vi "Resize Image (Scale).vi"(7 "Filter (Default)":T1, 8 "error in (no error)":errorcluster, 10 "Scale":dbl=1.0, 11 "Image":T2) -> (0 "error out":errorcluster, 3 "Resized Image":T2)   [LabVIEW 2020, in "G-Image.lvlib"]
doc: "Resize the input image by the specified scale multiplier.\n\n<b>Filter</b> sets the filter type used when resizing. When set to Default, the Catmull-Rom filter is used when upsampling images, and the Mitchell filter used when downsampling images.\n\n<b>Note:</b> 8-bit images will be converted to true color images when resized."
uses:
  G-Image.lvlib
  <vilib>/picture/picture.llb/imagedata.ctl
  Controls/Resize Filter.ctl
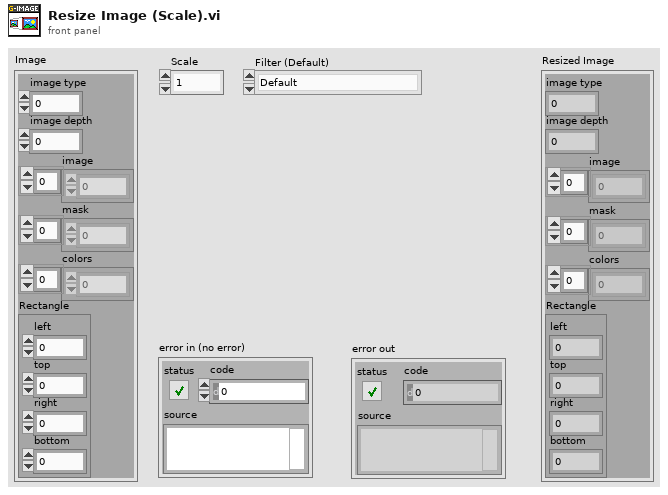
[diagram p1: front panel]
types:
  T1 = typedef "G-Image.lvlib/Resize Filter.ctl" = enum16{"Default", "Box", "Triangle", "Cubic B-Spline", "Catmull-Rom", "Mitchell"}
  T2 = typedef "imagedata.ctl" = cluster{"image type":i32, "image depth":i32, "image":u8[], "mask":u8[], "colors":u32[], "Rectangle":cluster{"left":i16, "top":i16, "right":i16, "bottom":i16}}
  T3 = cluster{"left":i16, "top":i16, "right":i16, "bottom":i16}
  T4 = cluster{"left":dbl, "top":dbl, "right":dbl, "bottom":dbl}
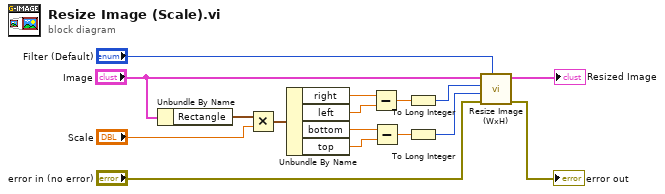
[diagram p0: block diagram]
diagram:
  n1 = Unbundle By Name("Image") -> ("Rectangle"=w16:T3)
  n2 = Multiply(x=w16, y="Scale") -> (x*y=w14:T4)
  n3 = Unbundle By Name(w14) -> ("right"=w13:dbl, "left"=w12:dbl, "bottom"=w9:dbl, "top"=w8:dbl)
  n4 = Subtract(x=w13, y=w12) -> (x-y=w11:dbl)
  n5 = Subtract(x=w9, y=w8) -> (x-y=w7:dbl)
  n6 = To Long Integer(number=w11) -> (32bit integer=w2:i32)
  n7 = To Long Integer(number=w7) -> (32bit integer=w1:i32)
  n8 = call "Resize Image (WxH).vi"("Filter (Default)"="Filter (Default)", "error in (no error)"="error in (no error)", "Height"=w1, "Width"=w2, "Image"="Image") -> ("error out"=→"error out":errorcluster, "Resized Image"=→"Resized Image":T2)  [unwired: 5 in]
